vi "Data to sumamry.vi"(5 "Window (ns)":i32, 7 "Period (seconds)":dbl, 9 "Trig lvl":string, 10 "ch2 data":i32[][](array[numeric]), 11 "ch1 data":i32[][](array[numeric])) -> (3 "String out":string)   [LabVIEW 2016]
uses:
  <vilib>/Analysis/NI_AALBase.lvlib
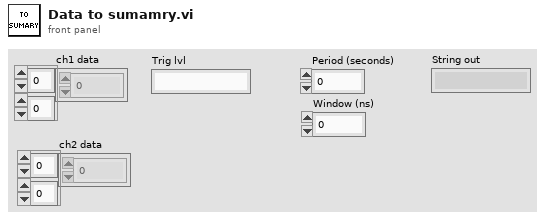
[diagram p1: front panel]
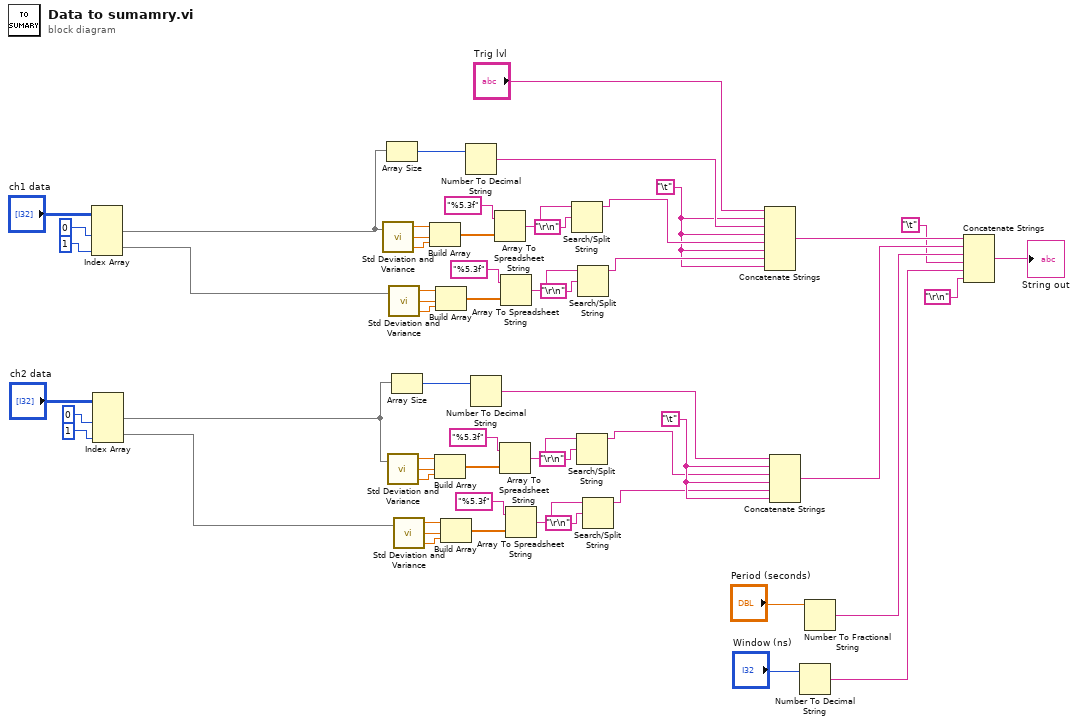
[diagram p0: block diagram]
diagram:
  w34 = "\t"
  w35 = "\t"
  n1 = Index Array(array="ch1 data", index (col) #1=0 ("index (row)"), index (col) #2=1 ("index (row)")) -> (element #1=w58:i32[], element #2=w37:i32[])  [unwired: 2 in]
  n2 = Index Array(array="ch2 data", index (col) #1=0 ("index (row)"), index (col) #2=1 ("index (row)")) -> (element #1=w15:i32[], element #2=w14:i32[])  [unwired: 2 in]
  n3 = call <vilib>:"Std Deviation and Variance.vi"("X"=w58) -> ("mean"=w53:dbl, "standard deviation"=w48:dbl, "variance"=w49:dbl)  [unwired: 1 in]
  n4 = Array Size(array=w58) -> (size(s)=w52:i32)
  n5 = call <vilib>:"Std Deviation and Variance.vi"("X"=w15) -> ("mean"=w19:dbl, "standard deviation"=w24:dbl, "variance"=w23:dbl)  [unwired: 1 in]
  n6 = call <vilib>:"Std Deviation and Variance.vi"("X"=w37) -> ("mean"=w40:dbl, "standard deviation"=w44:dbl, "variance"=w43:dbl)  [unwired: 1 in]
  n7 = Array Size(array=w15) -> (size(s)=w20:i32)
  n8 = call <vilib>:"Std Deviation and Variance.vi"("X"=w14) -> ("mean"=w30:dbl, "standard deviation"=w26:dbl, "variance"=w27:dbl)  [unwired: 1 in]
  n9 = Build Array(w53, w48, w49) -> (w51:dbl[])
  n10 = Build Array(w19, w24, w23) -> (w21:dbl[])
  n11 = Build Array(w40, w44, w43) -> (w41:dbl[])
  n12 = Build Array(w30, w26, w27) -> (w29:dbl[])
  n13 = Number To Decimal String(number=w52) -> (decimal integer string=w45:string)  [unwired: 1 in]
  n14 = Number To Decimal String(number=w20) -> (decimal integer string=w25:string)  [unwired: 1 in]
  n15 = Array To Spreadsheet String(array=w51, 3:"%5.3f" ("format string")) -> (spreadsheet string=w54:string)  [unwired: 1 in]
  n16 = Array To Spreadsheet String(array=w21, 3:"%5.3f" ("format string")) -> (spreadsheet string=w18:string)  [unwired: 1 in]
  n17 = Array To Spreadsheet String(array=w41, 3:"%5.3f" ("format string")) -> (spreadsheet string=w39:string)  [unwired: 1 in]
  n18 = Array To Spreadsheet String(array=w29, 3:"%5.3f" ("format string")) -> (spreadsheet string=w31:string)  [unwired: 1 in]
  n19 = Search/Split String(string=w54, search string/char (-)="\r\n") -> (substring before match=w56:string)  [unwired: 1 in, 2 out]
  n20 = Search/Split String(string=w18, search string/char (-)="\r\n") -> (substring before match=w16:string)  [unwired: 1 in, 2 out]
  n21 = Search/Split String(string=w39, search string/char (-)="\r\n") -> (substring before match=w36:string)  [unwired: 1 in, 2 out]
  n22 = Search/Split String(string=w31, search string/char (-)="\r\n") -> (substring before match=w33:string)  [unwired: 1 in, 2 out]
  n23 = Concatenate Strings("Trig lvl", w35, w45, w35, w56, w35, w36, w35) -> (w13:string)
  n24 = Concatenate Strings(w25, w34, w16, w34, w33, w34) -> (w12:string)
  n25 = Number To Decimal String(number="Window (ns)") -> (decimal integer string=w7:string)  [unwired: 1 in]
  n26 = Number To Fractional String(number="Period (seconds)") -> (F-format string=w9:string)  [unwired: 3 in]
  n27 = Concatenate Strings(w13, w12, w9, "\t", w7, "\r\n") -> (→"String out":string)
